vi "udp read.vi"() -> ()   [LabVIEW 2011]
panel:
  out "string":string[][](array[string]) caption="DateTime, IP, NMEA String"
  in  "Refresh Settings":bool
  in  "# hour per file":u16=1 min=1 max=24 step=1
  in  "Location":string="Unknown" caption="Location ID"
  in  "Save directory":path
  out "stats":string[][](array[string]) caption="DateTime,                 IP,                            Port(Hyd ID),         NMEA String"
  out "Packets":bool
  in  "IP":string caption="IP (leave blank)"
  in  "Timeout (50 ms)":i32
  in  "Service Name (leave blank)":string
  in  "port":u16 caption="Port (8040)"
  in  "Shutdown":bool
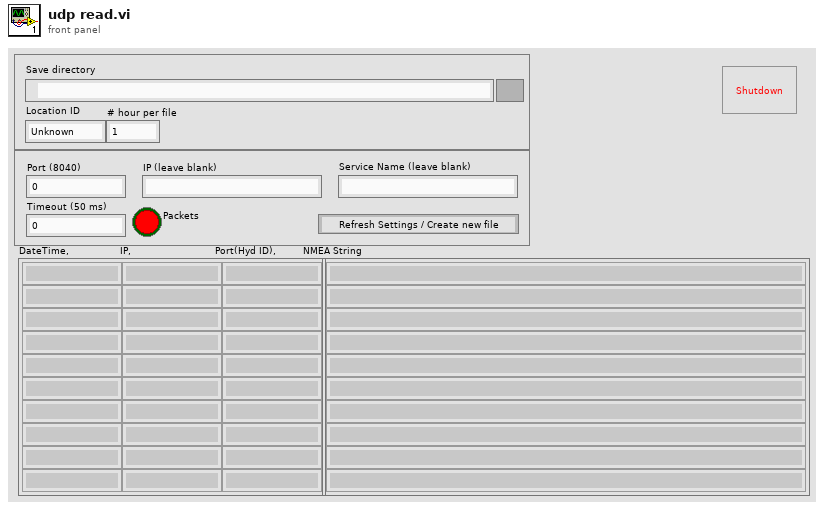
[diagram p1: front panel]
types:
  T1 = enum16{"big-endian, network order", "native, host order", "little-endian"}
  T2 = cluster{"IP":string, "port":u16, "service name":string, "timeout ms":i32, "Location":string, "Save directory":path, "# hour per file":u16}
  T3 = cluster{"IP":string, "port":u16, "Service Name (leave blank)":string, "Timeout (50 ms)":i32, "Location":string, "Save directory":path, "# hour per file":u16}
  T4 = enum32{"invalid app kind", "Development System", "Run Time System", "Student Edition", "Embedded LabVIEW", "Evaluation", "Custom"}
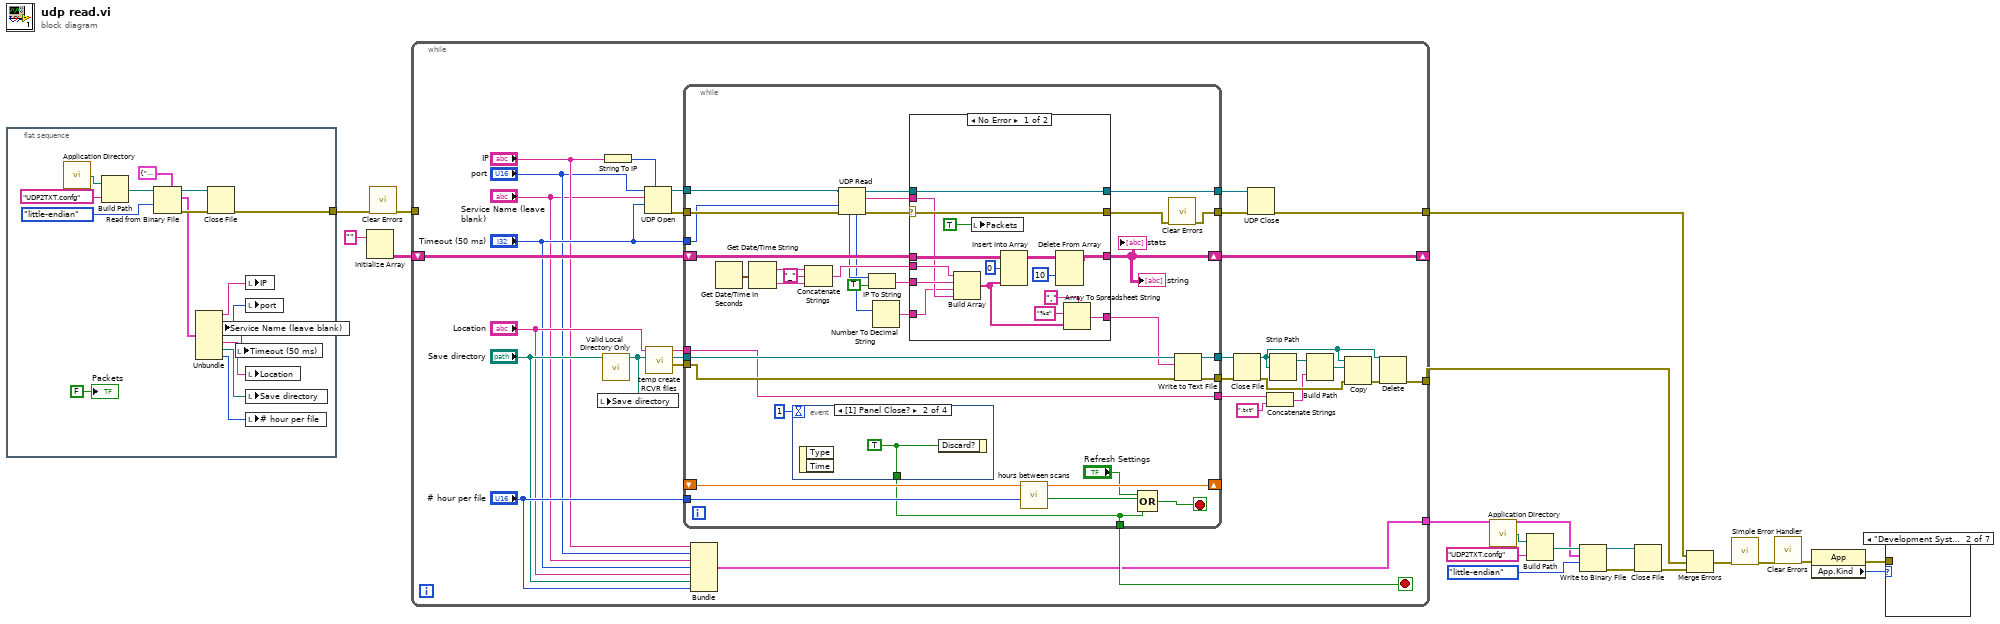
[diagram p0: block diagram]
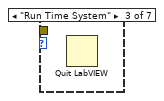
[diagram p3: hidden frame]
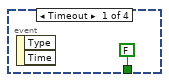
[diagram p8: hidden frame]
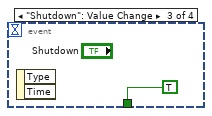
[diagram p9: hidden frame]
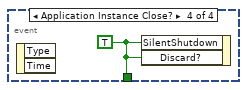
[diagram p10: hidden frame]
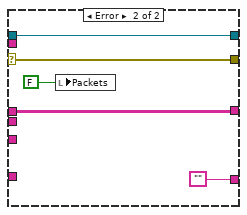
[diagram p11: hidden frame]
diagram:
  n1 = flat-sequence {
    tunnel: [w29] -> w2
    frame #0 {
      n2 = call <vilib>:"Application Directory.vi"() -> ("Application Directory"=w36:path)
      n3 = Build Path(base path=w36, name or relative path="UDP2TXT.confg") -> (appended path=w35:path)
      n4 = Read from Binary File(5:T2 {"IP"="", "port"=0, "service name"="", "timeout ms"=0, "Location"="", "Save directory"=path "", "# hour per file"=0}, 9:T1."little-endian" ("byte order (0:big-endian, network order)"), 11:w35) -> (0:w32:errorcluster, 2:w28:T2, 3:w33:refnum<file>)  [unwired: 3 in, 1 out]
      n5 = Unbundle(w28) -> ("IP"=w27:string, "port"=w26:u16, "service name"=w25:string, "timeout ms"=w24:i32, "Location"=w23:string, "Save directory"=w22:path, "# hour per file"=w21:u16)
      n6 = Close File(refnum=w33, error in=w32) -> (error out=w29:errorcluster)  [unwired: 1 out]
      n7 = local write "Service Name (leave blank)"(w25) -> ()
      n8 = local write "Timeout (50 ms)"(w24) -> ()
      n9 = local write "IP"(w27) -> ()
      n10 = local write "port"(w26) -> ()
      n11 = local write "Location"(w23) -> ()
      n12 = local write "Save directory"(w22) -> ()
      n13 = local write "# hour per file"(w21) -> ()
      "Packets" <- FALSE ("Packets")
    }
  }
  n14 = Initialize Array("") -> (w19:string[][])  [unwired: 2 in]
  n15 = call <vilib>:"Clear Errors.vi"("error in (no error)"=w2) -> ("error out"=w1:errorcluster)  [unwired: 6 in]
  n16 = while {
    tunnel: [w38] -> w4
    shift-right: [w67] -> _
    shift-left: w19 -> [w68]
    tunnel: w1 -> [_]
    tunnel: [w48] -> w8
    tunnel: [w47] -> w5
    stop <- w66 stop-if-true
    n17 = call "Valid Local Directory Only.vi"("Path input"="Save directory") -> ("Path output"=w52:path)  [unwired: 9 in, 1 out]
    n18 = local write "Save directory"(w52) -> ()
    n19 = String To IP(1:"IP") -> (0:w42:u32)
    n20 = UDP Open(7:w42, 9:"Timeout (50 ms)", 10:"Service Name (leave blank)", 11:"port") -> (port=w46:refnum<k16>, 0:w45:errorcluster)  [unwired: 1 in, 1 out]
    n21 = call "temp create RCVR files.vi"("Base File Path"=w52, "Location"="Location") -> ("error out"=w64:errorcluster, "refnum out"=w65:refnum<file>, "Name of file out"=w54:string)  [unwired: 7 in]
    n22 = while {
      tunnel: [w74] -> w66
      tunnel: w65 -> [w91]
      tunnel: w64 -> [w90]
      tunnel: [w88] -> w56
      tunnel: [w87] -> w55
      tunnel: w54 -> [w86]
      tunnel: [w86] -> w53
      shift-right: [w69] -> w67
      shift-left: w68 -> [w103]
      shift-right: [w84] -> _
      shift-left: _ -> [w83]
      tunnel: "# hour per file" -> [w82]
      tunnel: w46 -> [w80]
      tunnel: w45 -> [w79]
      tunnel: "Timeout (50 ms)" -> [w78]
      tunnel: [w76] -> w39
      tunnel: [w77] -> w37
      stop <- w92 stop-if-true
      n23 = Get Date/Time In Seconds() -> (seconds since 1Jan1904=w97:timestamp)
      n24 = Get Date/Time String(seconds (now)=w97) -> (date string=w96:string, time string=w95:string)  [unwired: 2 in]
      n25 = event shown="[1] Panel Close?" {
        selector: _ -> [_ _ _ _]
        dyn-events: _ -> [_ _ _ _]
        timeout: 1 -> [_ _ _ _]
        tunnel: [FALSE ("SilentShutdown") w105 TRUE w107] -> w74
        event Timeout {
          n26 = event-data() -> ()  [unwired: 1 in, 2 out]
        }
        event Panel Close? {
          w105 = TRUE ("Discard?")
          n27 = event-data() -> ()  [unwired: 1 in, 2 out]
          n28 = event-data("Discard?"=w105) -> ()  [unwired: 1 in, 1 out]
        }
        event "Shutdown": Value Change {
          n29 = event-data() -> ()  [unwired: 1 in, 2 out]
        }
        event Application Instance Close? {
          w107 = TRUE ("SilentShutdown")
          n30 = event-data() -> ()  [unwired: 1 in, 2 out]
          n31 = event-data("SilentShutdown"=w107, "Discard?"=w107) -> ()  [unwired: 1 in, 1 out]
        }
      }
      n32 = Concatenate Strings(w96, "_" ("string"), w95) -> (w93:string)
      n33 = UDP Read(connection ID=w80, timeout ms (25000)=w78, 8:w79) -> (data out=w102:string, error out=w101:errorcluster, 3:w99:refnum<k16>, 4:w71:u16, 6:w72:u32)  [unwired: 1 in]
      n34 = IP To String(1:TRUE ("dot notation? (F)"), 2:w72) -> (0:w98:string)
      n35 = Number To Decimal String(number=w71) -> (decimal integer string=w70:string)  [unwired: 1 in]
      n36 = case shown="No Error" w101 {
        selector: w101 -> [w122 w127]
        tunnel: w103 -> [w123 w128]
        tunnel: w102 -> [w109 _]
        tunnel: [w119 w128] -> w69
        tunnel: [w122 w127] -> w75
        tunnel: w99 -> [w120 w126]
        tunnel: [w120 w126] -> w77
        tunnel: w98 -> [w115 _]
        tunnel: w93 -> [w114 _]
        tunnel: [w111 ""] -> w89
        tunnel: w70 -> [w108 _]
        frame No Error {
          n37 = Build Array(w114, w115, w108, w109) -> (w112:string[])
          n38 = local write "Packets"(TRUE ("No packets")) -> ()
          n39 = Insert Into Array(array=w123, index (row)=0 ("index"), new element=w112) -> (w116:string[][])  [unwired: 1 in]
          n40 = Delete From Array(array=w116, index (row)=10 ("index")) -> (array with subset deleted=w119:string[][])  [unwired: 2 in, 1 out]
          n41 = Array To Spreadsheet String(delimiter (Tab)=",", array=w112, 3:"%s" ("format string")) -> (spreadsheet string=w111:string)
        }
        frame Error {
          n42 = local write "Packets"(FALSE ("No packets")) -> ()
        }
      }
      "stats" <- w69
      "string" <- w69
      n43 = call "hours between scans.vi"("Number of hours To Collect before starting new file"=w82, "Input start time"=w83) -> ("Time has Elapsed"=w85:bool, "output next start time"=w84:dbl)  [unwired: 7 in, 1 out]
      n44 = Compound Arithmetic op=OR("Refresh Settings", w85, w74) -> (w92:bool)
      n45 = call <vilib>:"Clear Errors.vi"("error in (no error)"=w75) -> ("error out"=w76:errorcluster)  [unwired: 6 in]
      n46 = Write to Text File(file (use dialog)=w91, text=w89, error in=w90) -> (refnum out=w88:refnum<file>, error out=w87:errorcluster)  [unwired: 1 in, 1 out]
    }
    n47 = Bundle("IP"="IP", "port"="port", "Service Name (leave blank)"="Service Name (leave blank)", "Timeout (50 ms)"="Timeout (50 ms)", "Location"="Location", "Save directory"="Save directory", "# hour per file"="# hour per file") -> (w48:T3)  [unwired: 1 in]
    n48 = Close File(refnum=w56, error in=w55) -> (path=w59:path, error out=w60:errorcluster)
    n49 = UDP Close(connection ID=w37, 8:w39) -> (error out=w38:errorcluster)  [unwired: 1 out]
    n50 = Concatenate Strings(w53, ".txt" ("string")) -> (w57:string)
    n51 = Strip Path(path=w59) -> (stripped path=w62:path)  [unwired: 1 out]
    n52 = Build Path(base path=w62, name or relative path=w57) -> (appended path=w63:path)
    n53 = Copy(8:w60, 10:w63, 11:w59) -> (0:w61:errorcluster)  [unwired: 2 in, 2 out]
    n54 = Delete(path (use dialog)=w59, error in=w61) -> (error out=w47:errorcluster)  [unwired: 3 in, 2 out]
  }
  n55 = call <vilib>:"Application Directory.vi"() -> ("Application Directory"=w7:path)
  n56 = Build Path(base path=w7, name or relative path="UDP2TXT.confg") -> (appended path=w10:path)
  n57 = Write to Binary File(file (use dialog)=w10, data=w8, 9:T1."little-endian" ("byte order (0:big-endian, network order)")) -> (refnum out=w12:refnum<file>, error out=w13:errorcluster)  [unwired: 3 in, 1 out]
  n58 = Close File(refnum=w12, error in=w13) -> (error out=w6:errorcluster)  [unwired: 1 out]
  n59 = Merge Errors(w4, w5, w6) -> (w3:errorcluster)
  n60 = call <vilib>:"Simple Error Handler.vi"("error in (no error)"=w3) -> ("error out"=w15:errorcluster)  [unwired: 4 in, 4 out]
  n61 = call <vilib>:"Clear Errors.vi"("error in (no error)"=w15) -> ("error out"=w9:errorcluster)  [unwired: 6 in]
  n62 = property class="App"(error in=w9) -> (error out=w17:errorcluster, "App.Kind"=w16:T4)  [unwired: 1 in, 1 out]
  n63 = case shown="\"Development System\"" w16 {
    tunnel: w17 -> [_ _ _ _ _ _ _]
    frame "invalid app kind", Default {
    }
    frame "Development System" {
    }
    frame "Run Time System" {
      n64 = Quit LabVIEW() -> ()  [unwired: 1 in]
    }
    frame "Student Edition" {
    }
    frame "Embedded LabVIEW" {
    }
    frame "Evaluation" {
    }
    frame "Custom" {
    }
  }
